vi "Gaussian Olasılık Fonk.vi"() -> ()   [LabVIEW 2015]
uses:
  <vilib>/gmath/NI_Gmath.lvlib
  <vilib>/Utility/file.llb/Read Delimited Spreadsheet (DBL).vi
  <vilib>/gmath/statdist.llb/Normal CDF.vi
panel:
  out "Waveform Chart":dbl(graph)
  out "Veriler":dbl[][](array[numeric])
  in  "Okunacak Veri Adresi":path
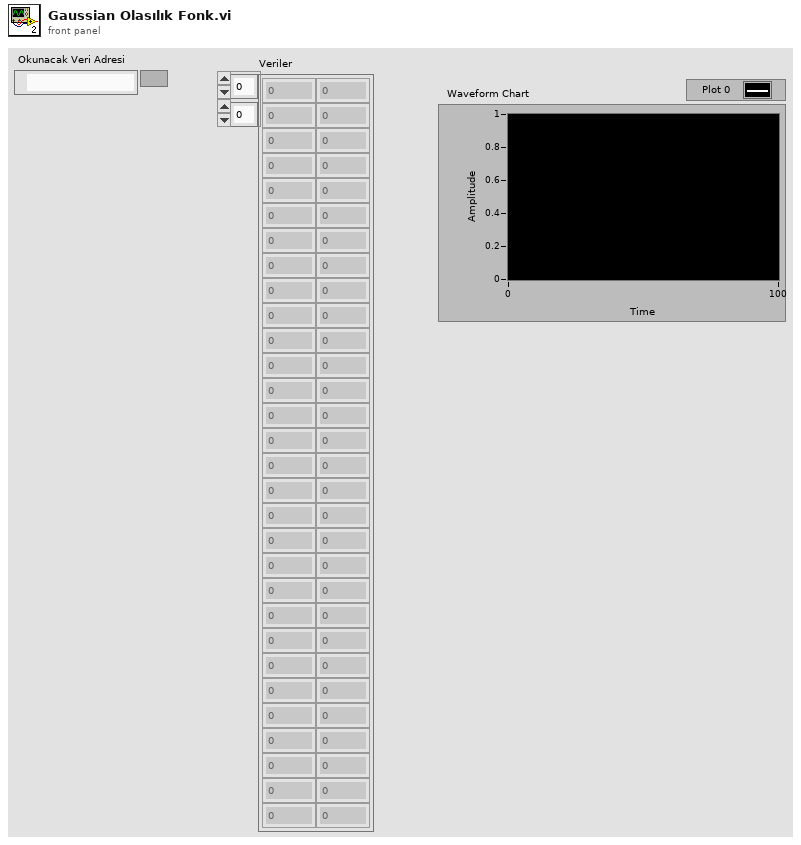
[diagram p1: front panel]
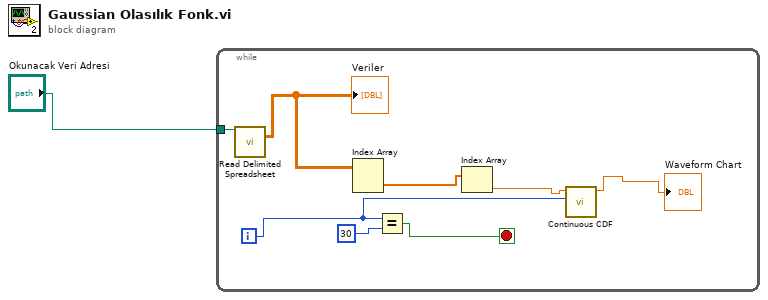
[diagram p0: block diagram]
diagram:
  n1 = while {
    tunnel: "Okunacak Veri Adresi" -> [w3]
    i -> [w2]
    stop <- w8 stop-if-true
    n2 = call-poly <vilib>:"Read Delimited Spreadsheet.vi"("file path (dialog if empty)"=w3) -> ("all rows"=w4:dbl[][])  [unwired: 9 in, 5 out]
    "Veriler" <- w4
    n3 = Index Array(array=w4) -> (element=w5:dbl[])  [unwired: 2 in]
    n4 = Equal?(x=w2, y=30) -> (x = y?=w8:bool)
    n5 = Index Array(array=w5) -> (element=w7:dbl)  [unwired: 1 in]
    n6 = call-poly <vilib>:"Continuous CDF.vi"("mean"=w2, "x"=w7) -> ("cdf(x)"=→"Waveform Chart":dbl)  [unwired: 8 in, 1 out]
  }
